vi "MyRICommandAndResponse.vi"(8 "error in (no error)":errorcluster, 9 "Min byte count":u32, 10 "Command":string="READ:SYS:USER", 11 "VISA resource name in":refnum<visa-resource-name>="TCPIP0::192.168.0.107::33576::SOCKET") -> (0 "error out":errorcluster, 2 "Response":string, 3 "VISA resource name out":refnum<visa-resource-name>)   [LabVIEW 2025, in "MyTriton.lvlib"]
uses:
  MyTriton.lvlib
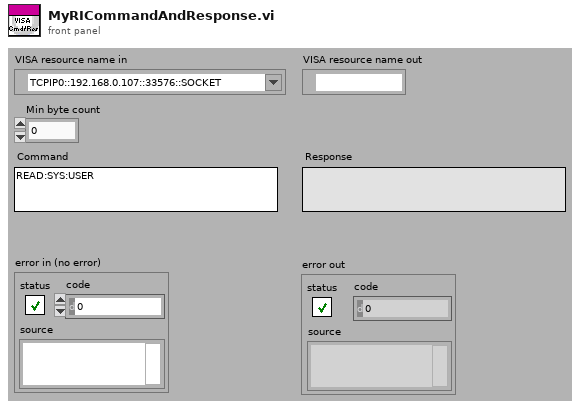
[diagram p1: front panel]
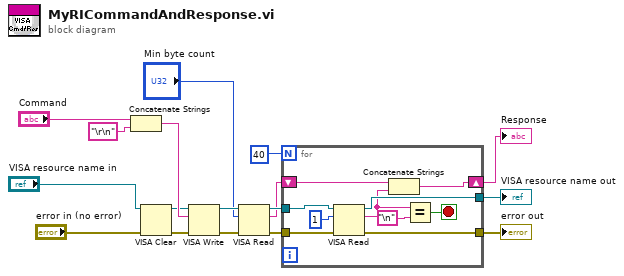
[diagram p0: block diagram]
diagram:
  n1 = Concatenate Strings("Command", "\r\n" ("string")) -> (w16:string)
  n2 = VISA Clear(VISA resource name="VISA resource name in", error in (no error)="error in (no error)") -> (VISA resource name out=w10:refnum<visa-resource-name>, error out=w9:errorcluster)
  n3 = VISA Write(VISA resource name=w10, write buffer=w16, error in (no error)=w9) -> (VISA resource name out=w8:refnum<visa-resource-name>, error out=w5:errorcluster)  [unwired: 1 out]
  n4 = VISA Read(VISA resource name=w8, byte count="Min byte count", error in (no error)=w5) -> (VISA resource name out=w7:refnum<visa-resource-name>, read buffer=w4:string, error out=w6:errorcluster)  [unwired: 1 out]
  n5 = for {
    N: 40 -> [_]
    tunnel: w7 -> [w26]
    tunnel: w6 -> [w25]
    tunnel: [w24] -> w3
    tunnel: [w23] -> w17
    shift-right: [w22] -> w2
    shift-left: w4 -> [w21]
    stop <- w19 stop-if-true
    n6 = VISA Read(VISA resource name=w26, byte count=u32 1, error in (no error)=w25) -> (VISA resource name out=w23:refnum<visa-resource-name>, read buffer=w20:string, error out=w24:errorcluster)  [unwired: 1 out]
    n7 = Concatenate Strings(w21, w20) -> (w22:string)
    n8 = Equal?(x=w20, y="\n") -> (x = y?=w19:bool)
  }
  "error out" <- w3
  "VISA resource name out" <- w17
  "Response" <- w2
